vi "Close Module.vi"(8 "error in (no error)":errorcluster, 9 "Wait for stop?":bool, 11 "Module Admin in":refnum<class "Delacor_lib_QMH_Cloneable Module Admin.lvclass">) -> (0 "error out":errorcluster, 1 "External Launch":bool, 3 "Module Admin out":refnum<class "Delacor_lib_QMH_Cloneable Module Admin.lvclass">)   [LabVIEW 2014, in "DB_CONNECTOR.lvlib"]
doc: "Destroy the Broadcast Events and Request Events (if this was the first instance). Reset flags stored in Module Admin class.\n_____\nBased on Delacor QMH Project Template 4.0.0.43.\n\n<b>Note:</b> This VI was modified by the <b>Validate DQMH Module</b> tool to upgrade it to the DQMH 5.0 approach to destroying cloneable module event references."
uses:
  DB_CONNECTOR.lvlib
  <vilib>/Delacor/Delacor QMH/Libraries/Cloneable Module Admin_class/Delacor_lib_QMH_Cloneable Module Admin.lvclass
  <vilib>/Delacor/Delacor QMH/Libraries/Cloneable Module Admin_class/Delacor_lib_QMH_Cloneable Module Admin.lvclass/Delacor_lib_QMH_Cloneable Module Admin.ctl
  <vilib>/Delacor/Delacor QMH/Libraries/Module Admin_class/Delacor_lib_QMH_Module Admin.lvclass/Delacor_lib_QMH_Module Admin.ctl
  <vilib>/Delacor/Delacor QMH/Libraries/Cloneable Module Admin_class/Delacor_lib_QMH_Get First.vi
  <vilib>/Delacor/Delacor QMH/Libraries/Cloneable Module Admin_class/Delacor_lib_QMH_Get Module ID.vi
  <vilib>/Delacor/Delacor QMH/Libraries/Module Admin_class/Delacor_lib_QMH_Get External Launch.vi
  Clone Registration/Clone Registration.lvlib
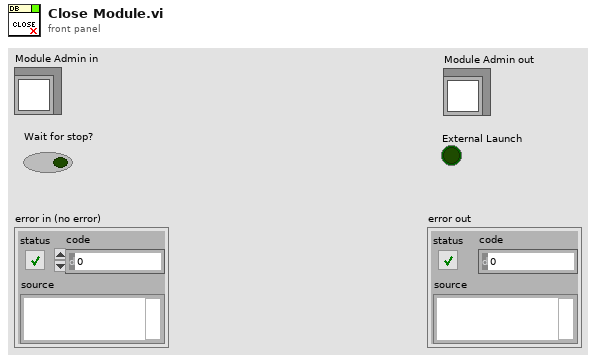
[diagram p1: front panel]
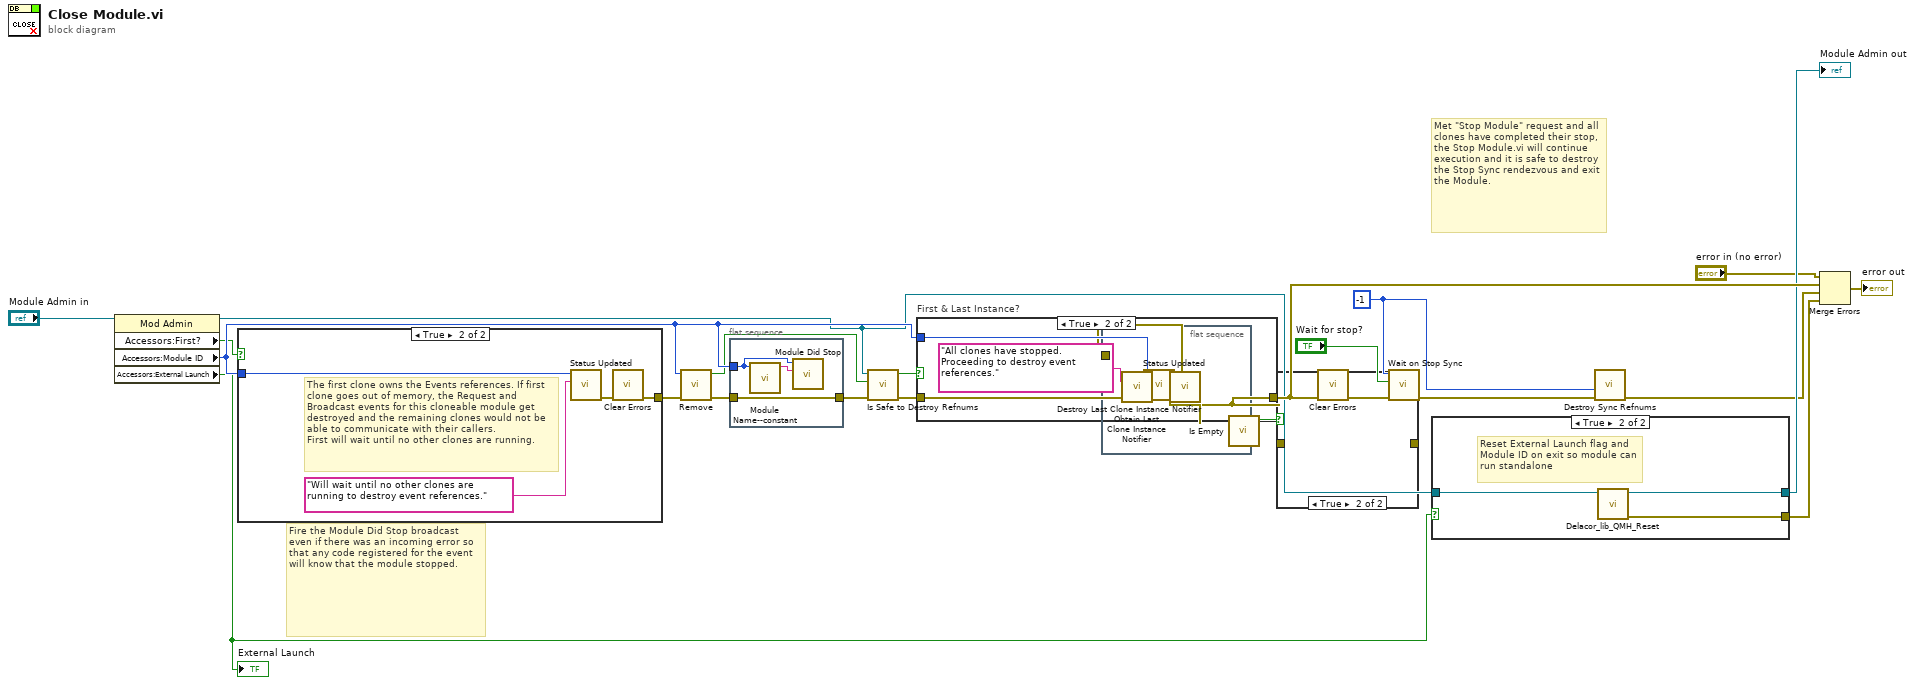
[diagram p0: block diagram]
diagram:
  w8 = -1 ("Module ID")
  # "Fire the Module Did Stop broadcast even if there was an incoming error so that any code registered for the event will know that the module stopped."
  # "Met \"Stop Module\" request and all clones have completed their stop, the Stop Module.vi will continue execution and it is safe to destroy the Stop Sync rendezvous and exit the Module."
  n1 = property class="Mod Admin"(reference="Module Admin in") -> (reference out=w16:refnum<class "Delacor_lib_QMH_Cloneable Module Admin.lvclass">, "Accessors:First?"=w5:bool, "Accessors:Module ID"=w20:i32, "Accessors:External Launch"=w4:bool)  [unwired: 1 in, 1 out]
  "External Launch" <- w4
  n2 = case shown="True" w5 {
    tunnel: w20 -> [_ w24]
    tunnel: [_ w22] -> w21
    frame False {
    }
    frame True {
      # "The first clone owns the Events references. If first clone goes out of memory, the Request and Broadcast events for this cloneable module get destroyed and the remaining clones would not be able to communicate with their callers.\nFirst will wait until no other clones are running."
      n3 = call "Status Updated.vi"("Status"="Will wait until no other clones are running to destroy event references." ("format string"), "Module ID"=w24) -> ("error out"=w23:errorcluster)  [unwired: 9 in]
      n4 = call <vilib>:"Clear Errors.vi"("error in (no error)"=w23) -> ("error out"=w22:errorcluster)  [unwired: 5 in, 1 out]
    }
  }
  n5 = call "Remove.vi"("error in (no error)"=w21, "Module ID"=w20) -> ("error out"=w17:errorcluster, "empty"=w2:bool)  [unwired: 7 in, 1 out]
  n6 = flat-sequence {
    tunnel: w17 -> [w28]
    tunnel: [w28] -> w1
    tunnel: w20 -> [w26]
    frame #0 {
      n7 = call "Module Name--constant.vi"("Module ID"=w26) -> ("Module Name"=w27:string)  [unwired: 10 in]
      n8 = call "Module Did Stop.vi"("Origin"=w27, "Module ID"=w26) -> ()  [unwired: 9 in, 1 out]
    }
  }
  n9 = call "Is Safe to Destroy Refnums.vi"("error in (no error)"=w1, "empty"=w2, "Module Admin"=w16) -> ("error out"=w13:errorcluster, "Destroy Broadcast & Request Event Refs?"=w14:bool)  [unwired: 7 in]
  n10 = case "First & Last Instance?" shown="True" w14 {
    tunnel: w13 -> [w29 w36]
    tunnel: [w29 w32] -> w19
    tunnel: w20 -> [_ w35]
    frame False {
    }
    frame True {
      n11 = flat-sequence {
        tunnel: w32 -> [_]
        frame #0 {
          n12 = call "Obtain Last Clone Instance Notifier.vi"() -> ("Last Instance Notifier"=w41:refnum<notifier>)  [unwired: 10 in, 1 out]
          n13 = call "Destroy Last Clone Instance Notifier.vi"("Last Instance Notifier"=w41) -> ()  [unwired: 11 in]
        }
      }
      n14 = call "Status Updated.vi"("error in (no error)"=w36, "Status"="All clones have stopped. Proceeding to destroy event references.", "Module ID"=w35) -> ("error out"=w33:errorcluster)  [unwired: 8 in]
      n15 = call "Is Empty.vi"("error in (no error)"=w33) -> ("error out"=w30:errorcluster, "Empty?"=w31:bool)  [unwired: 9 in]
      n16 = case shown="True" w31 {
        tunnel: w30 -> [w37 w40]
        tunnel: [w37 w38] -> w32
        frame False {
        }
        frame True {
          n17 = call "Destroy Broadcast Events.vi"("error in (no error)"=w40) -> ("error out"=w39:errorcluster)  [unwired: 10 in]
          n18 = call "Destroy Request Events.vi"("error in (no error)"=w39) -> ("error out"=w38:errorcluster)  [unwired: 10 in]
        }
      }
    }
  }
  n19 = call <vilib>:"Clear Errors.vi"("error in (no error)"=w19) -> ("error out"=w7:errorcluster)  [unwired: 5 in, 1 out]
  n20 = call "Wait on Stop Sync.vi"("error in (no error)"=w7, "Wait for Module to stop?"="Wait for stop?", "Module ID"=w8) -> ("error out"=w11:errorcluster)  [unwired: 8 in]
  n21 = case shown="True" w4 {
    tunnel: w16 -> [w42 w45]
    tunnel: [w42 w44] -> w12
    tunnel: [_ w43] -> w18
    frame False {
    }
    frame True {
      # "Reset External Launch flag and Module ID on exit so module can run standalone"
      n22 = call-dynamic "Delacor_lib_QMH_Reset.vi"("Mod Admin in"=w45) -> ("error out"=w43:errorcluster, "Mod Admin out"=w44:refnum<class "Delacor_lib_QMH_Cloneable Module Admin.lvclass">)  [unwired: 9 in]
    }
  }
  "Module Admin out" <- w12
  n23 = call "Destroy Sync Refnums.vi"("error in (no error)"=w11, "Module ID"=w8) -> ("error out"=w9:errorcluster)  [unwired: 9 in]
  n24 = Merge Errors("error in (no error)", w19, w9, w18) -> (→"error out":errorcluster)
